vi "Add Message Channel.vi"(8 "error in (no error)":errorcluster, 10 "Message Name":string, 11 "Message Group in":u64) -> (0 "error out":errorcluster, 1 "Message out":T1 format="%.0x", 3 "Message Group out":T1 format="%.0x")   [LabVIEW 2020, in "Instrument Addon Scripting API.lvlib"]
uses:
  Instrument Addon Scripting API.lvlib
  <vilib>/NI VeriStand/Custom Device API/Custom Device Item Ref.ctl
  Shared Directory/Constants.vi
  Shared Directory/Instrument Addon Shared.lvlib
  <vilib>/NI VeriStand/Custom Device API/Custom Device API.lvlib
  <vilib>/NI VeriStand/Custom Device Tools/Custom Device Utility Library/Custom Device Utility Library.lvlib
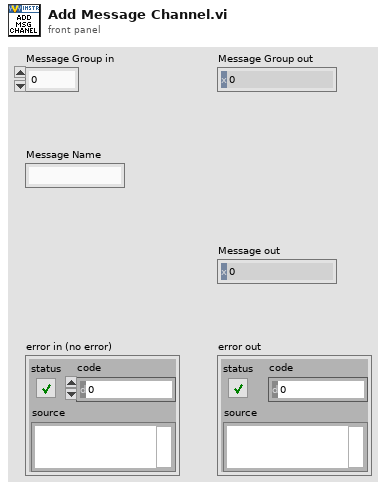
[diagram p1: front panel]
types:
  T1 = typedef "Custom Device API.lvlib/Custom Device Item Ref.ctl" = u64
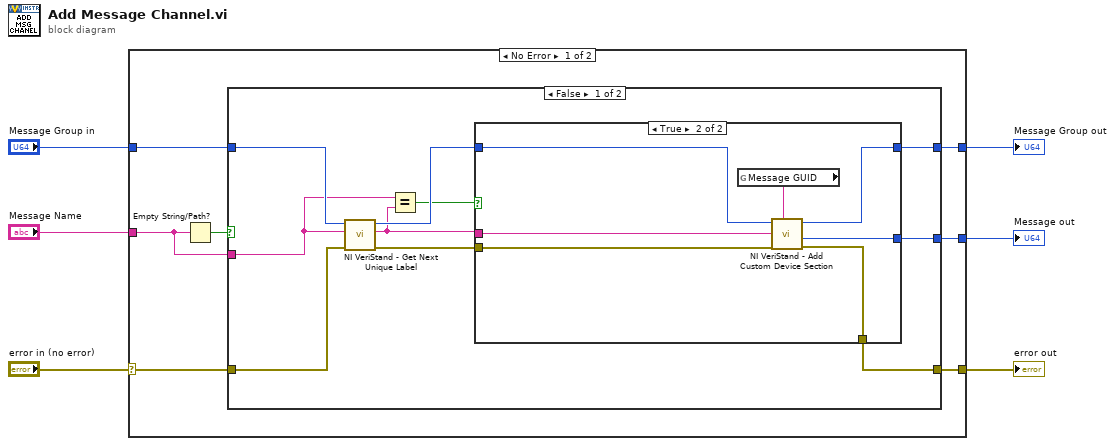
[diagram p0: block diagram]
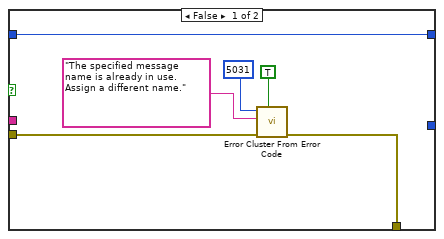
[diagram p2: hidden frame]
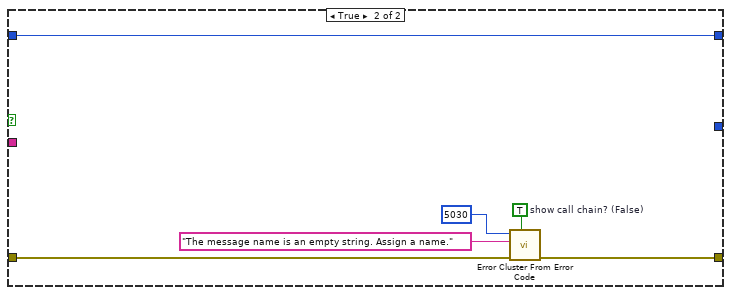
[diagram p3: hidden frame]
diagram:
  n1 = case shown="No Error" "error in (no error)" {
    selector: "error in (no error)" -> [w9 w44]
    tunnel: [w13 _] -> w6
    tunnel: [w12 w44] -> w5
    tunnel: [w11 w43] -> w4
    tunnel: "Message Name" -> [w7 _]
    tunnel: "Message Group in" -> [w10 w43]
    frame No Error {
      n2 = Empty String/Path?(string/path=w7) -> (empty?=w8:bool)
      n3 = case shown="False" w8 {
        tunnel: [w23 _] -> w13
        tunnel: [w22 w38] -> w12
        tunnel: [w21 w42] -> w11
        tunnel: w10 -> [w18 w42]
        tunnel: w9 -> [w17 w37]
        tunnel: w7 -> [w15 _]
        frame False {
          n4 = call <vilib>:"NI VeriStand - Get Next Unique Label.vi"("error in (no error)"=w17, "Label"=w15, "Parent Ref in"=w18) -> ("error out"=w20:errorcluster, "Label out"=w14:string, "Parent Ref dup"=w19:T1)  [unwired: 5 in, 1 out]
          n5 = Equal?(x=w15, y=w14) -> (x = y?=w16:bool)
          n6 = case shown="True" w16 {
            tunnel: [_ w36] -> w23
            tunnel: [w25 w35] -> w22
            tunnel: [w24 w33] -> w21
            tunnel: w20 -> [w26 w32]
            tunnel: w19 -> [w24 w31]
            tunnel: w14 -> [_ w30]
            frame False {
              n7 = call <vilib>:"Error Cluster From Error Code.vi"("show call chain? (False)"=TRUE, "error in (no error)"=w26, "error message (\"\")"="The specified message name is already in use. Assign a different name." ("error message (\"\")"), "error code (0)"=5031) -> ("error out"=w25:errorcluster)  [unwired: 5 in]
            }
            frame True {
              n8 = global read "Constants.vi" "Message GUID"() -> (w34:string)
              n9 = call <vilib>:"NI VeriStand - Add Custom Device Section.vi"("GUID (Default Section)"=w34, "error in (no error)"=w32, "Section Name"=w30, "Parent Ref in"=w31) -> ("error out"=w35:errorcluster, "Section Ptr"=w36:T1, "Parent Ref out"=w33:T1)  [unwired: 4 in, 1 out]
            }
          }
        }
        frame True {
          w39 = TRUE  # show call chain? (False)
          n10 = call <vilib>:"Error Cluster From Error Code.vi"("show call chain? (False)"=w39, "error in (no error)"=w37, "error message (\"\")"="The message name is an empty string. Assign a name." ("error message (\"\")"), "error code (0)"=5030) -> ("error out"=w38:errorcluster)  [unwired: 5 in]
        }
      }
    }
    frame Error {
    }
  }
  "Message out" <- w6
  "error out" <- w5
  "Message Group out" <- w4
